vi "DSF.Execution.Runtime.Plugin Manager.Check If Plugins Folder Exists.vi"(8 "error in (no error)":errorcluster, 11 "Plugin Manager in":refnum<class "DSF.Engine.Runtime.Plugin Manager.lvclass">) -> (0 "error out":errorcluster, 3 "Plugin Manager out":refnum<class "DSF.Engine.Runtime.Plugin Manager.lvclass">)   [LabVIEW 2016, in "DSF.Engine.lvlib" / "DSF.Engine.Runtime.Plugin Manager.lvclass"]
uses:
  DSF.Engine.Runtime.Plugin Manager.lvclass
  DSF.Engine.Runtime.Plugin Manager.lvclass/DSF.Engine.Runtime.Plugin Manager.ctl
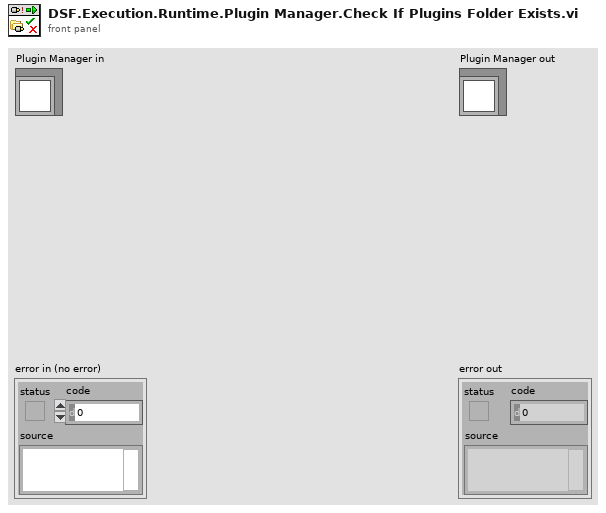
[diagram p1: front panel]
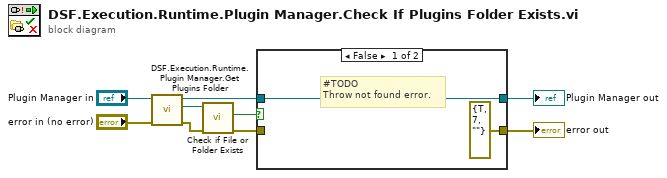
[diagram p0: block diagram]
diagram:
  n1 = call "DSF.Execution.Runtime.Plugin Manager.Get Plugins Folder.vi"("error in (no error)"="error in (no error)", "Plugin Manager in"="Plugin Manager in") -> ("error out"=w7:errorcluster, "Plugins folder"=w6:path, "Plugin Manager out"=w5:refnum<class "DSF.Engine.Runtime.Plugin Manager.lvclass">)  [unwired: 7 in]
  n2 = call <vilib>:"Check if File or Folder Exists.vi"("error in (no error)"=w7, "path"=w6) -> ("error out"=w2:errorcluster, "file or folder exists?"=w4:bool)  [unwired: 7 in, 1 out]
  n3 = case shown="False" w4 {
    tunnel: w5 -> [w11 w13]
    tunnel: [errorcluster {"status"=TRUE, "code"=7, "source"=""} ("error out") w12] -> w3
    tunnel: w2 -> [_ w12]
    tunnel: [w11 w13] -> w1
    frame False {
      # "#TODO\nThrow not found error."
    }
    frame True {
    }
  }
  "error out" <- w3
  "Plugin Manager out" <- w1
